vi "Create motor old.vi"(5 "max position":string, 6 "mech config":T1, 7 "max param":string, 8 "error in (no error)":errorcluster, 9 "name":string, 10 "id":string, 11 "Motor in":refnum<class "Motor.lvclass">) -> (0 "error out":errorcluster, 3 "Motor out":refnum<class "Motor.lvclass">)   [LabVIEW 2018, in "Motor.lvclass"]
uses:
  Motor.lvclass
  StateManager/StateManager.lvclass
  StateManager/StateManager.lvclass/StateManager.ctl
  Motor.lvclass/Motor.ctl
  MotorSim/MotorSim.lvclass
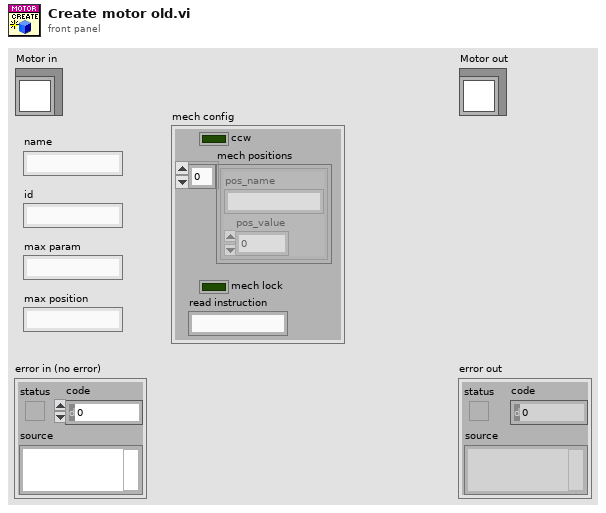
[diagram p1: front panel]
types:
  T1 = cluster{"ccw":bool, "mech positions":cluster{"pos_name":string, "pos_value":dbl}[], "mech lock":bool, "read instruction":string}
  T2 = cluster{"mode":string, "condition":string, "position":string, "pos_name":string, "pos_id":string}
  T3 = cluster{"period":u32, "initial position (0)":i32, "translation (100)":i32, "forward":bool}[]
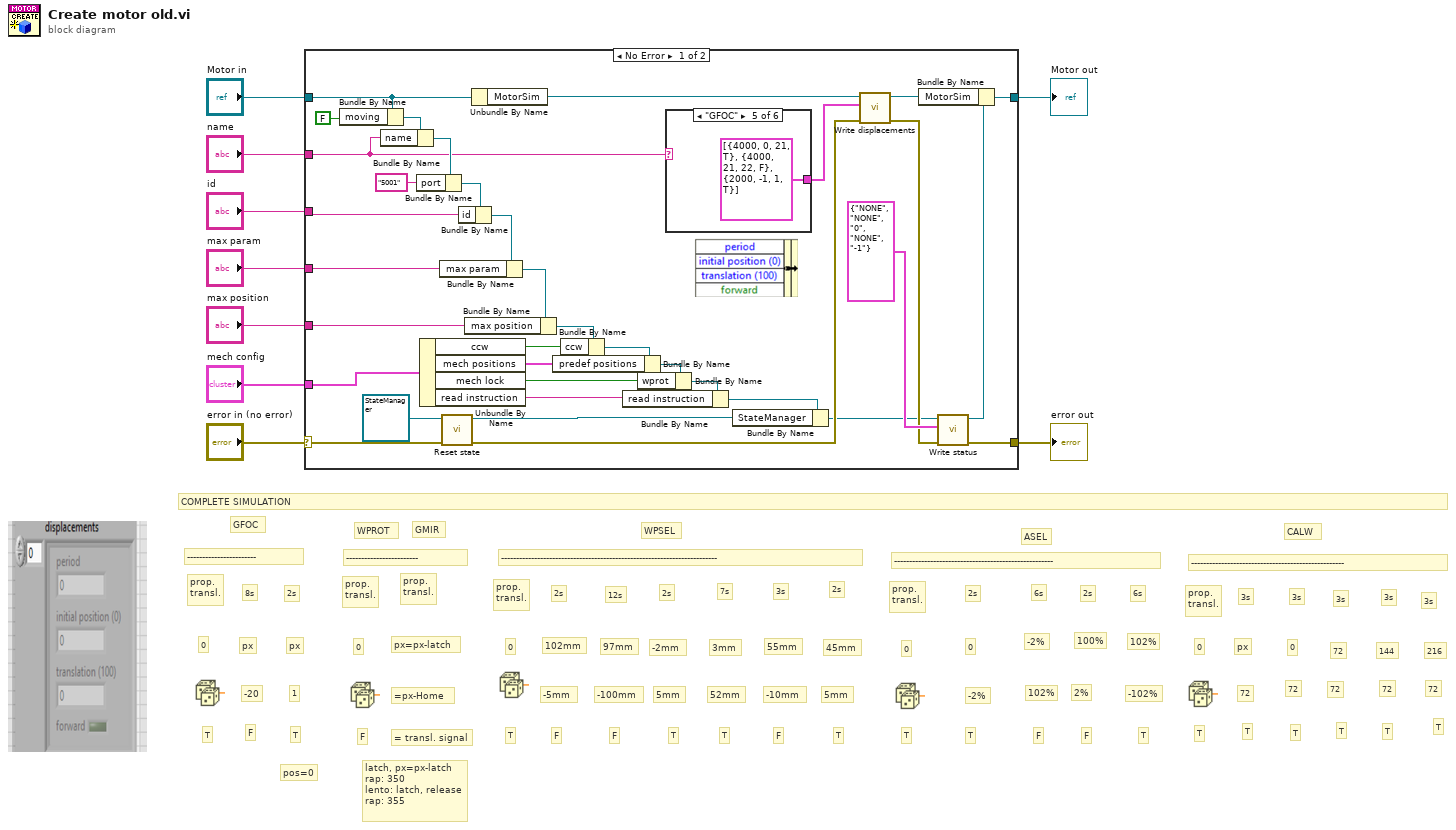
[diagram p0: block diagram]
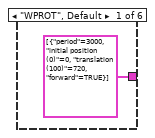
[diagram p2: hidden frame]
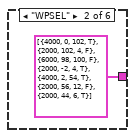
[diagram p3: hidden frame]
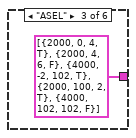
[diagram p4: hidden frame]
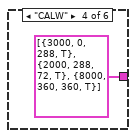
[diagram p5: hidden frame]
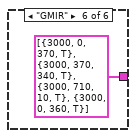
[diagram p6: hidden frame]
diagram:
  # "latch, px=px-latch\nrap: 350\nlento: latch, release\nrap: 355"
  # "COMPLETE SIMULATION"
  # "pos=0"
  # "1"
  # "px"
  # "T"
  # "2s"
  # "8s"
  # "-20"
  # "px"
  # "F"
  # "prop. \ntransl."
  # "T"
  # "0"
  # "-----------------------"
  # "GFOC"
  # "---------------------------------------------------"
  # "216"
  # "3s"
  # "T"
  # "72"
  # "144"
  # "72"
  # "0"
  # "72"
  # "72"
  # "72"
  # "3s"
  # "3s"
  # "3s"
  # "T"
  # "T"
  # "T"
  # "3s"
  # "T"
  # "72"
  # "px"
  # "prop. \ntransl."
  # "T"
  # "0"
  # "CALW"
  # "ASEL"
  # "-----------------------------------------------------"
  # "6s"
  # "T"
  # "-102%"
  # "102%"
  # "2s"
  # "F"
  # "2%"
  # "100%"
  # "102%"
  # "-2%"
  # "6s"
  # "F"
  # "-2%"
  # "2s"
  # "T"
  # "0"
  # "prop. \ntransl."
  # "T"
  # "0"
  # "------------------------"
  # "------------------------------------------------------------------------"
  # "T"
  # "5mm"
  # "45mm"
  # "2s"
  # "F"
  # "-10mm"
  # "55mm"
  # "3s"
  # "3mm"
  # "-2mm"
  # "52mm"
  # "7s"
  # "T"
  # "5mm"
  # "2s"
  # "T"
  # "prop. \ntransl."
  # "prop. \ntransl."
  # "prop. \ntransl."
  # "12s"
  # "97mm"
  # "F"
  # "-100mm"
  # "-5mm"
  # "2s"
  # "F"
  # "102mm"
  # "= transl. signal"
  # "px=px-latch"
  # "=px-Home"
  # "T"
  # "0"
  # "WPSEL"
  # "GMIR"
  # "F"
  # "0"
  # "WPROT"
  n1 = case shown="No Error" "error in (no error)" {
    selector: "error in (no error)" -> [w38 w51]
    tunnel: [w37 w51] -> w8
    tunnel: [w33 w52] -> w6
    tunnel: "Motor in" -> [w31 w52]
    tunnel: "name" -> [w32 _]
    tunnel: "id" -> [w44 _]
    tunnel: "max param" -> [w25 _]
    tunnel: "max position" -> [w21 _]
    tunnel: "mech config" -> [w20 _]
    frame No Error {
      n2 = Bundle By Name(cluster=w31, "moving"=FALSE) -> (w36:refnum<class "Motor.lvclass">)
      n3 = Bundle By Name(cluster=w36, "name"=w32) -> (w43:refnum<class "Motor.lvclass">)
      n4 = Bundle By Name(cluster=w43, "port"="5001") -> (w42:refnum<class "Motor.lvclass">)
      n5 = Unbundle By Name(w20) -> ("ccw"=w15:bool, "mech positions"=w14:cluster{"pos_name":string, "pos_value":dbl}[], "mech lock"=w19:bool, "read instruction"=w10:string)
      n6 = call "Reset state.vi"("error in (no error)"=w38, "StateManager in"=refnum<class "StateManager.lvclass"> refnum ("StateManager.lvclass")) -> ("error out"=w27:errorcluster, "StateManager out"=w40:refnum<class "StateManager.lvclass">)  [unwired: 8 in]
      n7 = Bundle By Name(cluster=w42, "id"=w44) -> (w23:refnum<class "Motor.lvclass">)
      n8 = Bundle By Name(cluster=w23, "max param"=w25) -> (w22:refnum<class "Motor.lvclass">)
      n9 = Bundle By Name(cluster=w22, "max position"=w21) -> (w18:refnum<class "Motor.lvclass">)
      n10 = Unbundle By Name(w31) -> ("MotorSim"=w29:refnum<class "MotorSim.lvclass">)
      n11 = Bundle By Name(cluster=w18, "ccw"=w15) -> (w17:refnum<class "Motor.lvclass">)
      n12 = Bundle By Name(cluster=w17, "predef positions"=w14) -> (w16:refnum<class "Motor.lvclass">)
      n13 = Bundle By Name(cluster=w16, "wprot"=w19) -> (w13:refnum<class "Motor.lvclass">)
      n14 = Bundle By Name(cluster=w13, "read instruction"=w10) -> (w12:refnum<class "Motor.lvclass">)
      n15 = case shown="\"GFOC\"" w32 {
        tunnel: [T3 [{"period"=3000, "initial position (0)"=0, "translation (100)"=720, "forward"=TRUE}] ("WPROT moves") T3 [{"period"=4000, "initial position (0)"=0, "translation (100)"=102, "forward"=TRUE}, {"period"=2000, "initial position (0)"=102, "translation (100)"=4, "forward"=FALSE}, {"period"=6000, "initial position (0)"=98, "translation (100)"=100, "forward"=FALSE}, {"period"=2000, "initial position (0)"=-2, "translation (100)"=4, "forward"=TRUE}, {"period"=4000, "initial position (0)"=2, "translation (100)"=54, "forward"=TRUE}, {"period"=2000, "initial position (0)"=56, "translation (100)"=12, "forward"=FALSE}, {"period"=2000, "initial position (0)"=44, "translation (100)"=6, "forward"=TRUE}] ("WPSEL moves") T3 [{"period"=2000, "initial position (0)"=0, "translation (100)"=4, "forward"=TRUE}, {"period"=2000, "initial position (0)"=4, "translation (100)"=6, "forward"=FALSE}, {"period"=4000, "initial position (0)"=-2, "translation (100)"=102, "forward"=TRUE}, {"period"=2000, "initial position (0)"=100, "translation (100)"=2, "forward"=TRUE}, {"period"=4000, "initial position (0)"=102, "translation (100)"=102, "forward"=FALSE}] ("ASEL moves") T3 [{"period"=3000, "initial position (0)"=0, "translation (100)"=288, "forward"=TRUE}, {"period"=2000, "initial position (0)"=288, "translation (100)"=72, "forward"=TRUE}, {"period"=8000, "initial position (0)"=360, "translation (100)"=360, "forward"=TRUE}] ("CALW moves") T3 [{"period"=4000, "initial position (0)"=0, "translation (100)"=21, "forward"=TRUE}, {"period"=4000, "initial position (0)"=21, "translation (100)"=22, "forward"=FALSE}, {"period"=2000, "initial position (0)"=-1, "translation (100)"=1, "forward"=TRUE}] ("GFOC moves") T3 [{"period"=3000, "initial position (0)"=0, "translation (100)"=370, "forward"=TRUE}, {"period"=3000, "initial position (0)"=370, "translation (100)"=340, "forward"=TRUE}, {"period"=3000, "initial position (0)"=710, "translation (100)"=10, "forward"=TRUE}, {"period"=3000, "initial position (0)"=0, "translation (100)"=360, "forward"=TRUE}] ("WPROT moves")] -> w26
        frame "WPROT", Default {
        }
        frame "WPSEL" {
        }
        frame "ASEL" {
        }
        frame "CALW" {
        }
        frame "GFOC" {
        }
        frame "GMIR" {
        }
      }
      n16 = Bundle By Name(cluster=w12, "StateManager"=w40) -> (w11:refnum<class "Motor.lvclass">)
      n17 = call-dynamic "Write displacements.vi"("error in (no error)"=w27, "displacements"=w26, "MotorSim in"=w29) -> ("error out"=w28:errorcluster, "MotorSim out"=w30:refnum<class "MotorSim.lvclass">)  [unwired: 7 in]
      n18 = call-dynamic "Write status.vi"("error in (no error)"=w28, "status"=T2 {"mode"="NONE", "condition"="NONE", "position"="0", "pos_name"="NONE", "pos_id"="-1"}, "Motor in"=w11) -> ("error out"=w37:errorcluster, "Motor out"=w34:refnum<class "Motor.lvclass">)  [unwired: 7 in]
      n19 = Bundle By Name(cluster=w34, "MotorSim"=w30) -> (w33:refnum<class "Motor.lvclass">)
    }
    frame Error {
    }
  }
  "error out" <- w8
  "Motor out" <- w6
